vi "Filter Active Elves.vi"(0 "Elf Locations in":set{T1}(c389), 1 "Destination":T1, 2 "#Active Elves":i32=100) -> (3 "Elf Locations out":set{T1}(c389))   [LabVIEW 2020, in "AoC 2022.lvlib"]
uses:
  AoC 2022.lvlib
  Day 15 - Beacon Exclusion Zone/private/Location.ctl
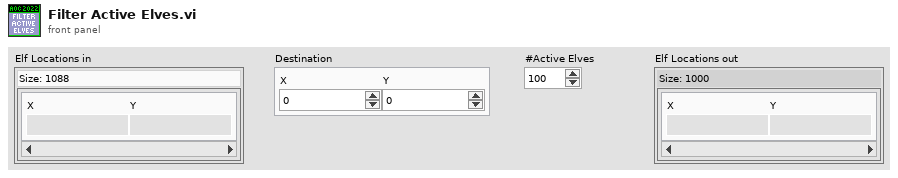
[diagram p1: front panel]
types:
  T1 = typedef "AoC 2022.lvlib/Location.ctl" = cluster{"X":i32, "Y":i32}
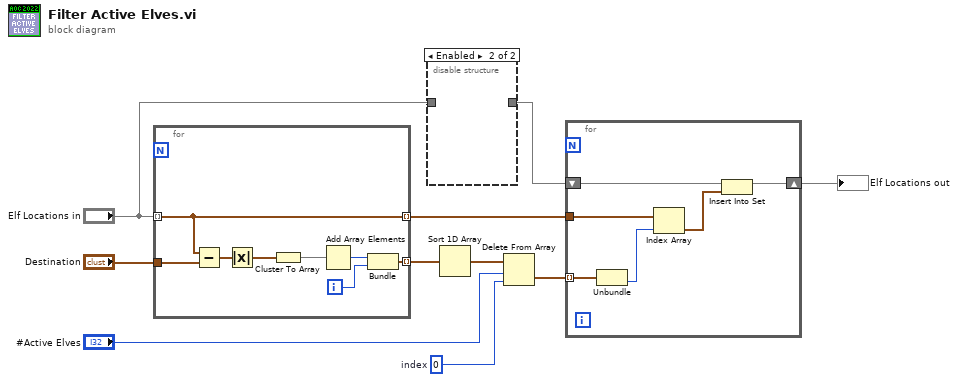
[diagram p0: block diagram]
diagram:
  w8 = 0  # index
  n1 = for {
    tunnel: "Elf Locations in" -> [w14] mode=indexing
    tunnel: "Destination" -> [w18]
    tunnel: [w14] -> w4 mode=indexing
    tunnel: [w11] -> w5 mode=indexing
    i -> [w12]
    n2 = Subtract(x=w14, y=w18) -> (x-y=w17:T1)
    n3 = Absolute Value(x=w17) -> (abs(x)=w16:T1)
    n4 = Cluster To Array(cluster=w16) -> (array=w15:i32[])
    n5 = Add Array Elements(numeric array=w15) -> (sum=w13:i32)
    n6 = Bundle("X"=w13, w12) -> (w11:cluster{"X":i32, i32})  [unwired: 1 in]
  }
  n7 = disable-structure shown="Enabled" {
    disable-tunnel: "Elf Locations in" -> [w19 _]
    disable-tunnel: [w19 _] -> w2
    frame Disabled {
    }
    frame Enabled {
    }
  }
  n8 = Sort 1D Array(array=w5) -> (sorted array=w6:cluster{"X":i32, i32}[])
  n9 = Delete From Array(array=w6, length="#Active Elves", index=w8) -> (deleted portion=w7:cluster{"X":i32, i32}[])  [unwired: 1 out]
  n10 = for {
    tunnel: w7 -> [w23] mode=indexing
    tunnel: w4 -> [w22]
    shift-right: [w24] -> w1
    shift-left: w2 -> [w25]
    n11 = Unbundle(w23) -> (w20:i32)  [unwired: 1 out]
    n12 = Index Array(array=w22, index=w20) -> (element=w21:T1)
    n13 = Insert Into Set(10:w21, 11:w25) -> (3:w24:set{T1})  [unwired: 1 out]
  }
  "Elf Locations out" <- w1
